vi "UIMsg Callback.vi"(5 "Callback ID":i32, 7 "Owner":refnum<class>, 10 "User Data":variant, 11 "UIMessage":refnum<class "UIMessage.lvclass">) -> (0 "error out":errorcluster)   [LabVIEW 2020, in "TSnax UI.lvlib" / "SequenceViewPanel.lvclass"]
uses:
  SequenceViewPanel.lvclass
  TSnax/UIMessage/UIMessage.lvclass
  SequenceViewPanel.lvclass/SequenceViewPanel.ctl
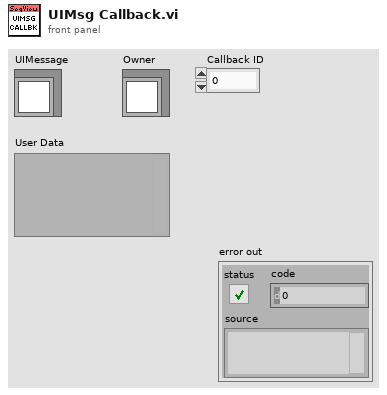
[diagram p1: front panel]
types:
  T1 = typedef "TSnax.lvlib/UIMsg.ctl" = enum16{"Unknown", "BreakOnUserRequest", "BreakOnBreakpoint", "BreakOnRunTimeError", "Trace", "TerminatingExecution", "AbortingExecution", "KillingExecutionThreads", "EndExecution", "ShutDownComplete", "StartExecution", "ProgressPercent", "ProgressText", "StartInteractiveExecution", "EndInteractiveExecution", "TerminatingInteractiveExecution", "TerminationCancelled", "ResumeFromBreak", "StartFileExecution", "EndFileExecution", "ShutDownCancelled", "LocalizationSettingChanged", "OpenWindows", "TileWindows", "CascadeWindows", "ReportChanged", "CloseWindows", "RefreshWindows", "ClientFileChanged", "DisplayReport", "ModelState_Initializing", "ModelState_Waiting", "ModelState_Identified", "ModelState_BeginTesting", "ModelState_TestingComplete", "ModelState_PostProcessingComplete", "ModelState_EnabledStateSet", "ReportLocationChanged", "GotoLocation", "PushUndoItem", "OutputMessages", "TypePaletteFileListChanged", "NonTerminatingThreadsArePreventingTermination", "ModelState_PostProcessing", "ReportCollectionChanged", "RuntimeError"}
  T2 = typedef "TSnax UI.lvlib/SequenceViewPanel.lvclass/Ref Data.ctl" = cluster{"Insert Line":i32, "SequenceFile":refnum<class "SequenceFile.lvclass">, "Sequence":string, "Trace Marker":i32}
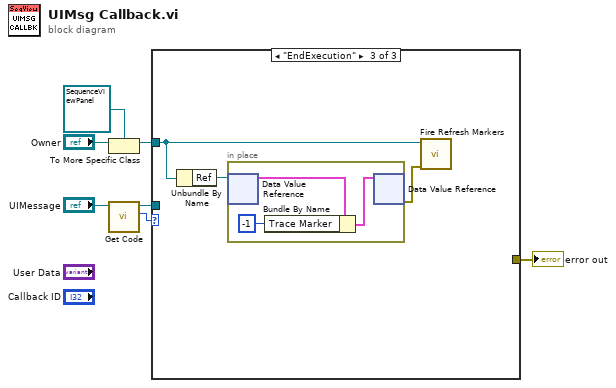
[diagram p0: block diagram]
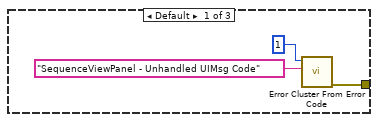
[diagram p2: hidden frame]
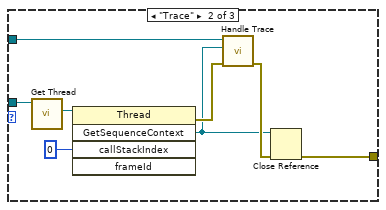
[diagram p3: hidden frame]
diagram:
  n1 = To More Specific Class(target class=refnum<class "SequenceViewPanel.lvclass"> refnum ("TSnax UI.lvlib:SequenceViewPanel.lvclass"), reference="Owner") -> (specific class reference=w3:refnum<class "SequenceViewPanel.lvclass">)  [unwired: 1 in, 1 out]
  n2 = call "Get Code.vi"("UIMessage in"="UIMessage") -> ("Code"=w4:T1, "UIMessage out"=w1:refnum<class "UIMessage.lvclass">)  [unwired: 8 in, 1 out]
  n3 = case shown="\"EndExecution\"" w4 {
    tunnel: w3 -> [_ w14 w20]
    tunnel: [w8 w11 _] -> w2
    tunnel: w1 -> [_ w16 _]
    frame Default {
      n4 = call <vilib>:"Error Cluster From Error Code.vi"("error message (\"\")"="SequenceViewPanel - Unhandled UIMsg Code" ("error message (\"\")"), "error code (0)"=1) -> ("error out"=w8:errorcluster)  [unwired: 7 in]
    }
    frame "Trace" {
      n5 = call "Get Thread.vi"("UIMessage in"=w16) -> ("Thread"=w15:refnum<k7>)  [unwired: 8 in, 2 out]
      n6 = invoke class="Thread" method="GetSequenceContext"(reference=w15, "callStackIndex"=0) -> (error out=w13:errorcluster, "GetSequenceContext"=w12:refnum<k7>)  [unwired: 3 in, 3 out]
      n7 = call "Handle Trace.vi"("error in (no error)"=w13, "Sequence Context"=w12, "SequenceViewPanel in"=w14) -> ("error out"=w18:errorcluster)  [unwired: 7 in, 1 out]
      n8 = Close Reference(reference=w12, error in (no error)=w18) -> (error out=w11:errorcluster)
    }
    frame "EndExecution" {
      n9 = Unbundle By Name(w20) -> ("Ref"=w21:refnum<data-value>)
      n10 = in-place {
        n11 = in-place-dvr #1(w21) -> (w24:T2)  [unwired: 1 out]
        n12 = Bundle By Name(cluster=w24, "Trace Marker"=-1) -> (w23:T2)
        n13 = in-place-dvr #1(w23) -> (w19:errorcluster)  [unwired: 1 out]
      }
      n14 = call "Fire Refresh Markers.vi"("error in (no error)"=w19, "SequenceViewPanel in"=w20) -> ()  [unwired: 8 in, 2 out]
    }
  }
  "error out" <- w2
